vi "SS_fpga_swept_sines_zaxis.vi"() -> ()   [LabVIEW 2017]
uses:
  controls/boolean_info.ctl
  subVIs/auto-sys-id/controls/sysID_control_params.ctl
  <vilib>/rvi/Emulation/niFpgaGetClockAttributes.vi
  <vilib>/rvi/Emulation/niFpgaSctlEmulationGetInTimedLoop.vi
  <vilib>/rvi/Emulation/niFpgaEmulationReportErrorSimple.vi
  <vilib>/rvi/eio/common/nirviEmuTemplateMethod_errors.vi
  <vilib>/rvi/Emulation/niFpgaCriticalErrorInLSC.vi
  <vilib>/rvi/Emulation/niFpgaProcessEmulError.vi
  <vilib>/eio/EIONode/EIONode.xnode
panel:
  in  "control-xy-zero":bool
  in  "Log-Channel_select":bool[](array[boolean])=[TRUE, TRUE, TRUE, TRUE, FALSE, FALSE]
  in  "Close Loop?":bool
  in  "Nsettle":u32
  in  "reset":bool=TRUE
  out "z-u(k)":sgl
  in  "DDS_params":T1={"Accumulator Increment"=100000, "Phase Shift"=0, "Signal Amplitude (x 2^15)"=32768}
  in  "ABORT":bool
  in  "Subtract y0?":bool
  in  "Swept-Sines-Control-Settings":T2={"u-max"=0.3, "offset"=0.0, "Ki"=0.001} {"offset" format="%#_4g"; "u-max" format="%#_13g"}
  out "iter":i32
  out "All Done":bool
  in  "TsTicks":u32=1600
  out "boolean \nindicators":T3
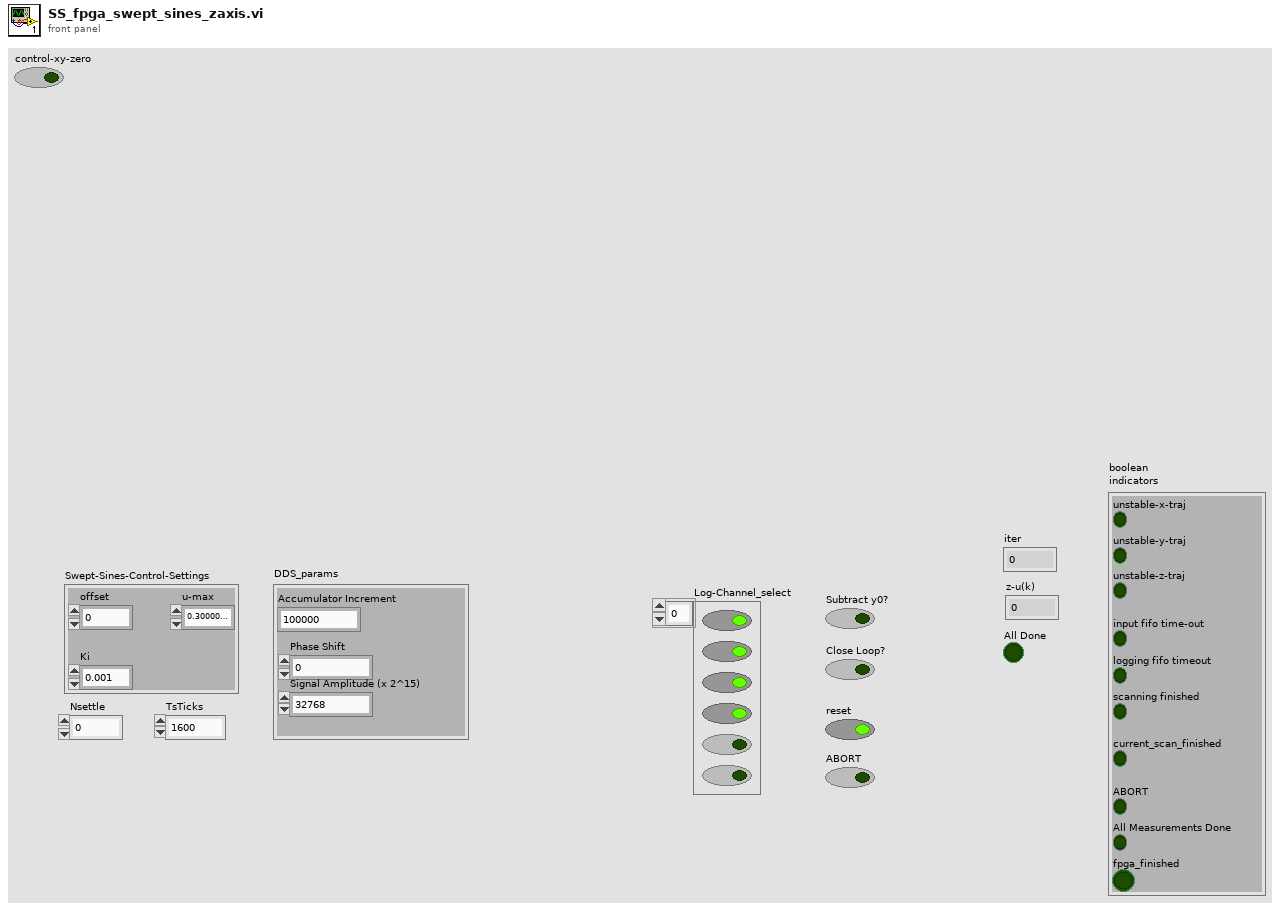
[diagram p1: front panel]
types:
  T1 = cluster{"Accumulator Increment":u32, "Phase Shift":u32, "Signal Amplitude (x 2^15)":u16}
  T2 = typedef "sysID_control_params.ctl" = cluster{"u-max":sgl, "offset":sgl, "Ki":sgl}
  T3 = typedef "boolean_info.ctl" = cluster{"unstable-z-traj":bool, "input fifo time-out":bool, "logging fifo timeout":bool, "scanning finished":bool, "unstable-x-traj":bool, "unstable-y-traj":bool, "ABORT":bool, "All Measurements Done":bool, "fpga_finished":bool, "current_scan_finished":bool}
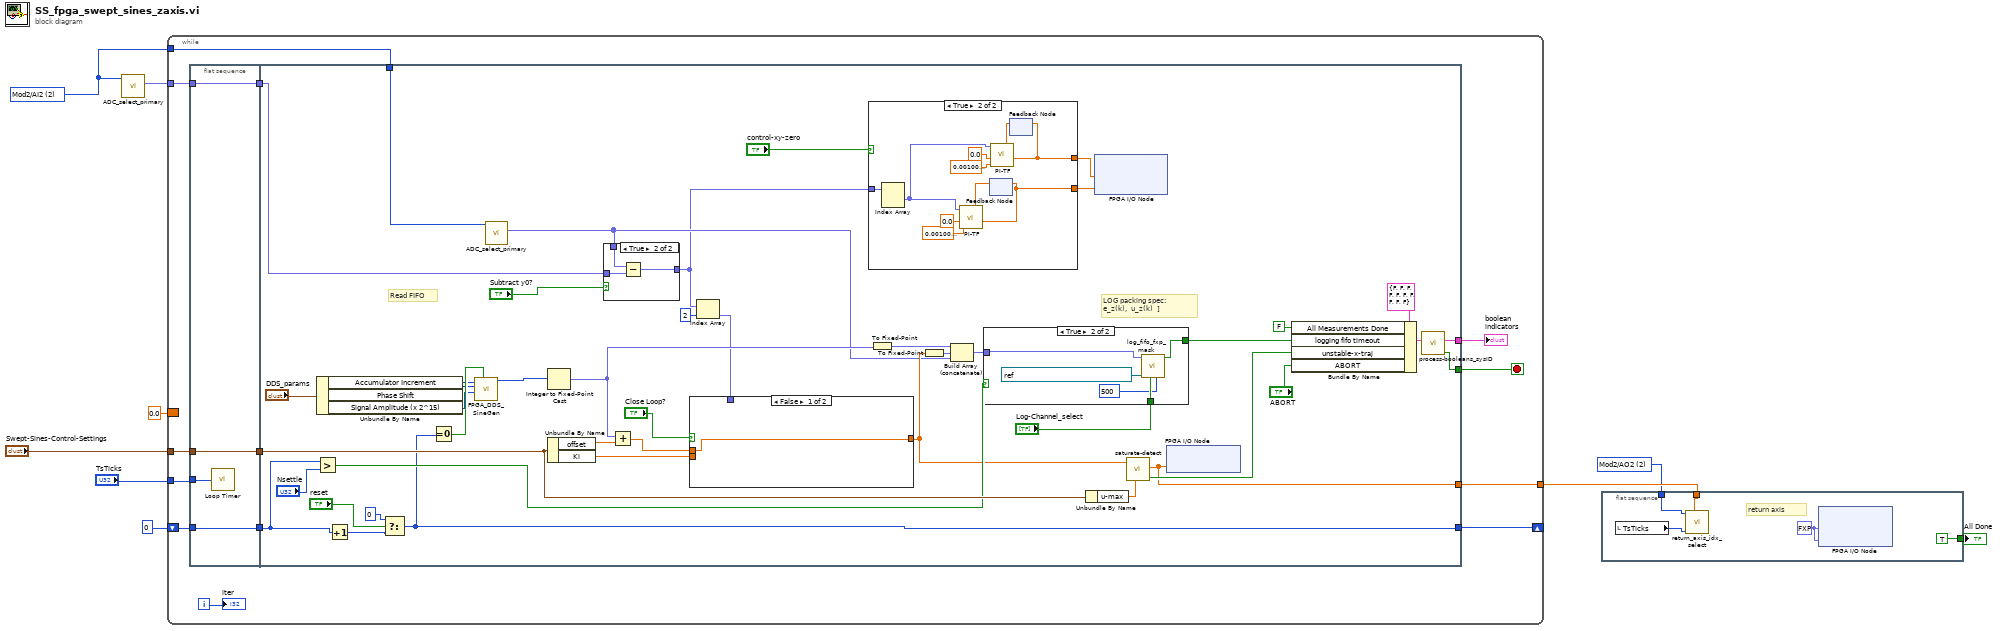
[diagram p0: block diagram]
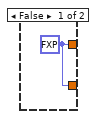
[diagram p2: hidden frame]
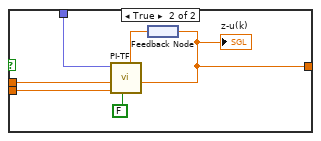
[diagram p3: hidden frame]
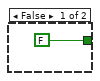
[diagram p5: hidden frame]
diagram:
  w3 = i16 2 items=["Mod2/AI0", "Mod2/AI1", "Mod2/AI2", "Mod2/AI3", ""] ("ADC-select")
  w1 = i16 2 items=["Mod2/AO0", "Mod2/AO1", "Mod2/AO2", "Mod2/AO3", ""] ("DAC-select")
  n1 = call "ADC_select_primary.vi"("ADC-primary-select"=w3) -> ("ADC-all"=w2:fxp<+/-,24,5>[])  [unwired: 9 in, 1 out]
  n2 = while {
    tunnel: "Swept-Sines-Control-Settings" -> [w21]
    tunnel: "TsTicks" -> [w20]
    tunnel: [w19] -> w8
    tunnel: w3 -> [w16]
    shift-right: [w13] -> _
    shift-left: u32 0 -> [w12]
    border: sgl 0.0 ("u(k)") -> [_]
    tunnel: w2 -> [w11]
    i -> [w15]
    stop <- w18 stop-if-true
    n3 = flat-sequence {
      tunnel: w20 -> [w25]
      tunnel: w21 -> [w26]
      tunnel: [w26] -> w22
      tunnel: [w24] -> w14
      tunnel: w12 -> [w24]
      tunnel: w11 -> [w23]
      tunnel: [w23] -> w10
      tunnel: w22 -> [w69]
      tunnel: [w28] -> w19
      tunnel: [w58] -> w18
      tunnel: [w57] -> w17
      tunnel: w16 -> [w37]
      tunnel: w14 -> [w45]
      tunnel: [w44] -> w13
      tunnel: w10 -> [w35]
      frame #0 {
        n4 = call "Loop Timer"("Count(Ticks)"=w25) -> ()  [unwired: 1 out]
      }
      frame #1 {
        # "LOG packing spec:\ne_z(k),  u_z(k)  ]"
        # "Read FIFO"
        n5 = Greater?(x=w45, y="Nsettle") -> (0:w50:bool)
        n6 = Unbundle By Name("DDS_params") -> ("Accumulator Increment"=w53:u32, "Phase Shift"=w52:u32, "Signal Amplitude (x 2^15)"=w51:u16)
        n7 = Increment(x=w45) -> (x+1=w49:u32)
        n8 = Select(t=u32 0, s="reset", f=w49) -> (s? t:f=w44:u32)
        n9 = Equal To 0?(x=w44) -> (x = 0?=w54:bool)
        n10 = call "FPGA_DDS_SineGen.vi"("Reset Accumulator"=w54, "Signal Amplitude (x 2^15)"=w51, "Phase Shift"=w52, "Accumulator Increment"=w53) -> ("Signal Value"=w55:i16)  [unwired: 6 in, 1 out]
        n11 = call "ADC_select_primary.vi"("ADC-primary-select"=w37) -> ("ADC-all"=w34:fxp<+/-,24,5>[])  [unwired: 9 in, 1 out]
        n12 = Unbundle By Name(w69) -> ("offset"=w66:sgl, "Ki"=w56:sgl)
        n13 = Integer to Fixed-Point Cast(integer=w55) -> (fixed-point=w39:fxp<+/-,16,5>)  [unwired: 1 in]
        n14 = case shown="True" "Subtract y0?" {
          tunnel: w35 -> [_ w91]
          tunnel: w34 -> [w89 w92]
          tunnel: [w89 w90] -> w33
          frame False {
          }
          frame True {
            n15 = Subtract(x=w92, y=w91) -> (x-y=w90:fxp<+/-,25,6>[])
          }
        }
        n16 = Add(x=w39, y=w66) -> (x+y=w67:sgl)
        n17 = Index Array(array=w33, index=2) -> (element=w31:fxp<+/-,25,6>)
        n18 = case shown="False" "Close Loop?" {
          tunnel: w67 -> [w82 w86]
          tunnel: w56 -> [_ w85]
          tunnel: w31 -> [_ w83]
          tunnel: [w82 w84] -> w41
          frame False {
          }
          frame True {
            n19 = feedback #1() -> (w88:sgl)
            n20 = call "PI-TF.vi"("u(k-1)"=w88, "reset"=FALSE, "Ki"=w85, "setpoint"=w86, "y(k)"=w83) -> ("u(k)"=w84:sgl)  [unwired: 6 in]
            "z-u(k)" <- w84
            n21 = feedback-in #1(w84) -> ()
          }
        }
        n22 = case shown="True" "control-xy-zero" {
          tunnel: w33 -> [_ w74]
          tunnel: [w71 w73] -> w30
          tunnel: [w71 w72] -> w29
          frame False {
            w71 = fxp<+,1,1> 0.0 ("u(k)")
          }
          frame True {
            n23 = Index Array(array=w74) -> (element #1=w75:fxp<+/-,25,6>)  [unwired: 2 in, 1 out]
            n24 = feedback #2() -> (w79:sgl)  [unwired: 1 in]
            n25 = call "PI-TF.vi"("u(k-1)"=w79, "Ki"=sgl 0.001, "setpoint"=sgl 0.0, "y(k)"=w75) -> ("u(k)"=w72:sgl)  [unwired: 7 in]
            n26 = feedback-in #2(w72) -> ()
            n27 = feedback #3() -> (w76:sgl)  [unwired: 1 in]
            n28 = call "PI-TF.vi"("u(k-1)"=w76, "Ki"=sgl 0.001, "setpoint"=sgl 0.0, "y(k)"=w75) -> ("u(k)"=w73:sgl)  [unwired: 7 in]
            n29 = feedback-in #3(w73) -> ()
          }
        }
        n30 = To Fixed-Point(number=w39) -> (fixed-point=w40:fxp<+/-,25,6>)  [unwired: 1 in]
        n31 = To Fixed-Point(number=w41) -> (fixed-point=w36:fxp<+/-,25,6>)  [unwired: 1 in]
        n32 = Build Array (concatenate)(w40, w36, w34) -> (w70:fxp<+/-,25,6>[])
        n33 = case shown="True" w50 {
          tunnel: w70 -> [_ w98]
          tunnel: [FALSE ("logging-timeout?") w97] -> w59
          tunnel: "Log-Channel_select" -> [_ w95]
          frame False {
          }
          frame True {
            n34 = call "log_fifo_fxp_mask.vi"("Timeout(ticks)"=500, "Log-Channel_select"=w95, "FIFO In"=refnum<k21> "fpga-to-host-fxp-16-5", "input-data"=w98) -> ("logging-timeout?"=w97:bool)  [unwired: 7 in]
          }
        }
        n35 = Unbundle By Name(w69) -> ("u-max"=w68:sgl)
        n36 = xnode "FPGA I/O Node"("Mod1/AO0"=w30, "Mod1/AO1"=w29) -> ()  [unwired: 2 in, 2 out]
        n37 = call "saturate-detect.vi"("bound"=w68, "x"=w41) -> ("saturated"=w60:bool, "sat(x)"=w28:sgl)  [unwired: 8 in]
        n38 = xnode "FPGA I/O Node"("Mod1/AO2"=w28) -> ()  [unwired: 1 in, 1 out]
        n39 = Bundle By Name(cluster=T3 {"unstable-z-traj"=FALSE, "input fifo time-out"=FALSE, "logging fifo timeout"=FALSE, "scanning finished"=FALSE, "unstable-x-traj"=FALSE, "unstable-y-traj"=FALSE, "ABORT"=FALSE, "All Measurements Done"=FALSE, "fpga_finished"=FALSE, "current_scan_finished"=FALSE} ("boolean errors"), "All Measurements Done"=FALSE, "logging fifo timeout"=w59, "unstable-x-traj"=w60, "ABORT"="ABORT") -> (w62:T3)
        n40 = call "process-booleans_sysID.vi"("boolean indicators 2"=w62) -> ("scaning finished"=w58:bool, "boolean indicators"=w57:T3)  [unwired: 9 in]
      }
    }
    "boolean \nindicators" <- w17
    "iter" <- w15
  }
  n41 = flat-sequence {
    tunnel: w8 -> [w102]
    tunnel: [TRUE] -> w7
    tunnel: w1 -> [w101]
    frame #0 {
      w99 = fxp<+/-,20,5> 0.0 ("Mod1/AO0")
      # "return axis"
      n42 = local read "TsTicks"() -> (w100:u32)
      n43 = call "return_axis_idx_select.vi"("u(0)"=w102, "TsTicks"=w100, "DAC-select"=w101) -> ()  [unwired: 9 in]
      n44 = xnode "FPGA I/O Node"("Mod1/AO0"=w99, "Mod1/AO1"=w99) -> ()  [unwired: 2 in, 2 out]
    }
  }
  "All Done" <- w7
